vi "uintPow.vi"(8 "Error in (no error)":errorcluster, 10 "Exponent":u32=2, 11 "Int in":refnum<class "UintClass.lvclass">) -> (0 "Error out":errorcluster, 1 "Timing":u32, 3 "pow(Int, Exponent)":refnum<class "UintClass.lvclass">)   [LabVIEW 2011, in "UintClass.lvclass"]
uses:
  UintClass.lvclass
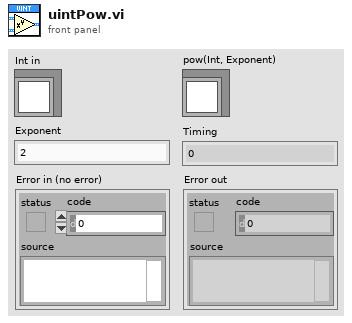
[diagram p1: front panel]
types:
  T1 = typedef "UintClass.lvclass/enumBase.ctl" = u16
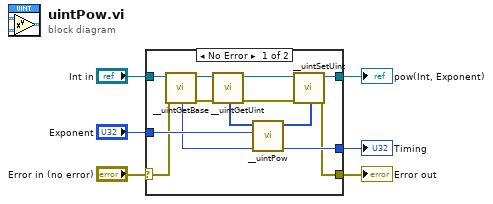
[diagram p0: block diagram]
diagram:
  n1 = case shown="No Error" "Error in (no error)" {
    selector: "Error in (no error)" -> [w14 w20]
    tunnel: "Int in" -> [w17 _]
    tunnel: "Exponent" -> [w18 _]
    tunnel: [w9 _] -> w3
    tunnel: [w8 _] -> w2
    tunnel: [w7 w20] -> w1
    frame No Error {
      n2 = call "__uintGetBase.vi"("Error in (no error)"=w14, "UintClass in"=w17) -> ("Error out"=w15:errorcluster, "Base (decimal)"=w13:T1, "UintClass out"=w16:refnum<class "UintClass.lvclass">)  [unwired: 7 in]
      n3 = call "__uintGetUint.vi"("Error in (no error)"=w15, "UintClass in"=w16) -> ("Error out"=w11:errorcluster, "Uint (0)"=w19:u8[], "UintClass out"=w12:refnum<class "UintClass.lvclass">)  [unwired: 7 in]
      n4 = call "__uintPow.vi"("Base (decimal)"=w13, "Exponent (2)"=w18, "UInt in"=w19) -> ("Timing multiplication"=w8:u32, "UInt^Exponent"=w10:u8[])  [unwired: 7 in]
      n5 = call "__uintSetUint.vi"("Error in (no error)"=w11, 10:"Uint in"=w10, 11:"Uint in"=w12) -> ("Error out"=w7:errorcluster, "Uint out"=w9:refnum<class "UintClass.lvclass">)  [unwired: 7 in]
    }
    frame Error {
    }
  }
  "Error out" <- w1
  "pow(Int, Exponent)" <- w3
  "Timing" <- w2
